vi "PDF Protokoll.vi"(8 "error in (no error)":errorcluster caption="Fehler (Eingang, kein Fehler)") -> (0 "error out":errorcluster caption="Fehler (Ausgang)")   [LabVIEW 2015, in "Linearisierung V2.lvlib" / "Protokoll.lvlib"]
uses:
  Protokoll.lvlib
  EPA Ausgabetabelle.ctl
  AktivArray.ctl
  AktivButton.ctl
  Aktion Lin Daten aufarbeiten.ctl
  EPA1065-307/Aktion FGV Auswertung sammeln.ctl
  <vilib>/Utility/miscctls.llb/LVPrintingMarginsTypeDef.ctl
  Linearisierung V2.lvlib
  EPA1065-307/Linearity verification 1065-307.lvlib
  Allgemein/allgemeine Sub-VIs.lvlib
  <vilib>/Utility/NIReport.llb/NI_ReportGenerationCore.lvlib
panel:
  out "XY-Graph EPA":cluster{dbl[], dbl[]}[](graph) caption="XY-Graph"
  out "Aktiv":T1
  out "EPA Ausgabetabelle":T3
  out "Ergebnis:":string
  out "Konzentration:":string
  out "Komponente:":string
  out "Bearbeiter:":string
  out "Gasteiler:":string
  out "Messgerät:":string
  out "EPA Auswertung":string[][](table) caption="Evaluation"
  # "Linearity Check EPA §1065.307"
  # "Linearity Check EPA § 1065.307"
  # "IAG-Industrie Automatisierungsgeschellschaft m.b.H.    l  Industriestraße 2    l    2722Weikersdorf     )+43262221734 7+43262221734655"
  # "Linearity detection §1065.307"
  # "Description of the limits"
  # "Slope (a1) value between 0,99-1,01"
  # "Intercept (a0)"
  # "laboratory: Value <= 0,5% of the gas concentration"
  # "field: Value <= 1% of the gas concentration"
  # "Coefficient of determination (R²) Value >= 0,998"
  # "standard error of estimate (SEE) Value <= 1% of the gas concentration"
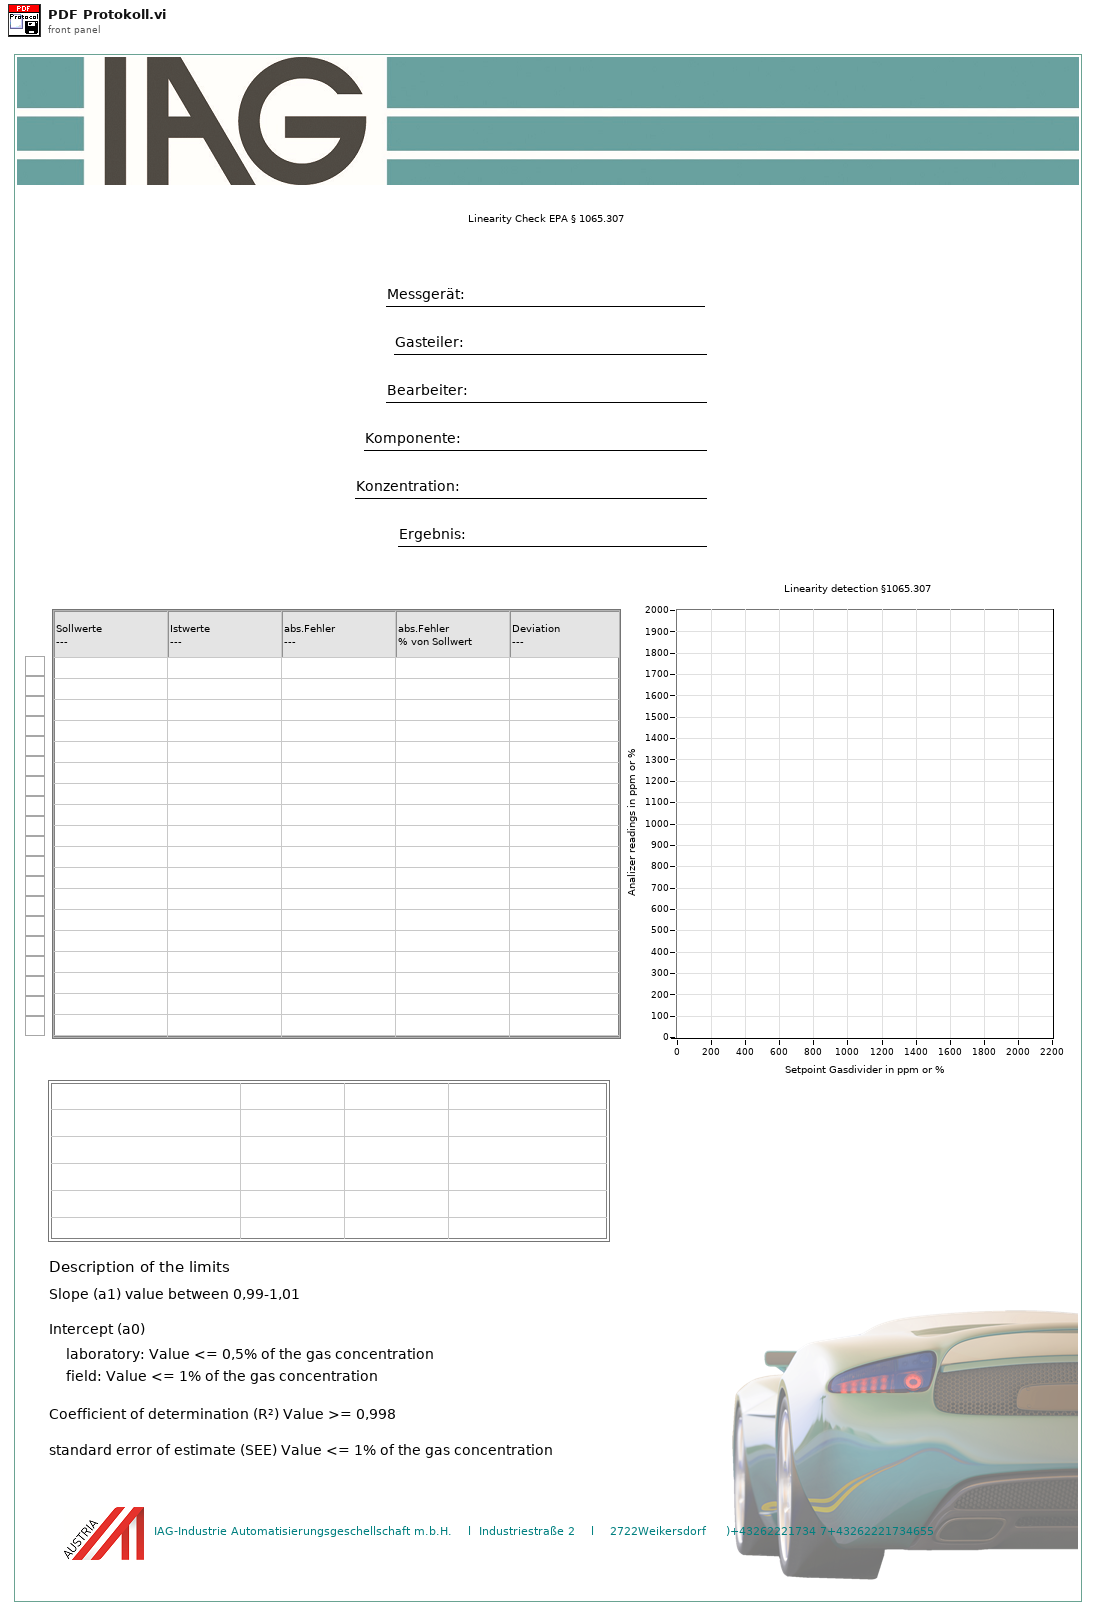
[diagram p1: front panel]
types:
  T1 = typedef "Linearisierung V2.lvlib/AktivArray.ctl" = T2[]
  T2 = typedef "Linearisierung V2.lvlib/AktivButton.ctl" = bool
  T3 = typedef "Linearisierung V2.lvlib/EPA Ausgabetabelle.ctl" = string[][]
  T4 = typedef "Linearisierung V2.lvlib/Aktion Lin Daten aufarbeiten.ctl" = enum16{"lesen", "Protkolldaten", "speichern", "laden", "EPA auswerten", "Tabelle schreiben", "Lin auswerten", "Tab init", "Stufentabelle", "EPA aktiviert", "Nachbehandlung laden", "Tabelle löschen", "Istwerte löschen", "Zeile löschen", "Zeile einfügen", "LIN aktiviert", "LIN/EPA aktiv laden"}
  T5 = typedef "Linearisierung V2.lvlib/Linearity verification 1065-307.lvlib/Aktion FGV Auswertung sammeln.ctl" = enum16{"lesen", "Auswertung", "löschen"}
  T6 = enum32{"Portrait", "Landscape", "Rotated Portrait", "Rotated Landscape"}
  T7 = typedef "LVPrintingMarginsTypeDef.ctl" = cluster{"Top":sgl, "Left":sgl, "Bottom":sgl, "Right":sgl, "Measurement System":enum8{"Inches", "cm"}}
  T8 = typedef "Auswahlfeld.ctl" = u16
  T9 = typedef "Linearisierung V2.lvlib/Eingabetabelle.ctl" = string[][]
  T10 = typedef "Linearisierung V2.lvlib/Lin-Polynom Daten.ctl" = cluster{"Messgerät":string, "Kalibrator (Gasteiler)":string, "Bearbeiter/in":string, "Komponente":string, "Zeitstempel":timestamp, "F_max gefordert (%)":sgl, "F_max in %":sgl, "F_max in ppm":sgl, "Vorschlag Ordnung":i32, "Polynom OK":bool, "Polynomkoeff.":sgl[], "Prüfgas Konzentration":sgl, "Pfad1":string, "Pfad_LIN":string, "Gasnummer:":u8, "Komponentenauswahl":T11, "Verdünnungsgas":T12, "Zeitdauer Stufe":T13, "Anzahl Stufen":T13, "F_max in % EPA":sgl, "F_max in ppm EPA":sgl, "F_max in % LIN":sgl, "F_max in ppm LIN":sgl, "Punkte umkehren":bool, "EPA Optionsfeld":T14, "Autolin Hovacal":T15}
  T11 = typedef "Linearisierung V2.lvlib/KomponentenArray.ctl" = cluster{"Komponente:":T8, "Konzentration":sgl}[]
  T12 = typedef "Linearisierung V2.lvlib/Gasteiler.lvlib/Prüfgas in.ctl" = u16
  T13 = typedef "Zahlen-Eingabefeld.ctl" = sgl
  T14 = typedef "Linearisierung V2.lvlib/EPA Optionsfeld.ctl" = enum32{"Istwert", "Rohwert", "Linearisierter Wert"}
  T15 = typedef "Linearisierung V2.lvlib/Gasteiler.lvlib/HovaCal.lvlib/AutoLin Hovacal.ctl" = enum32{"Keine Auswahl", "Optionsauswahl 1", "Optionsauswahl 2"}
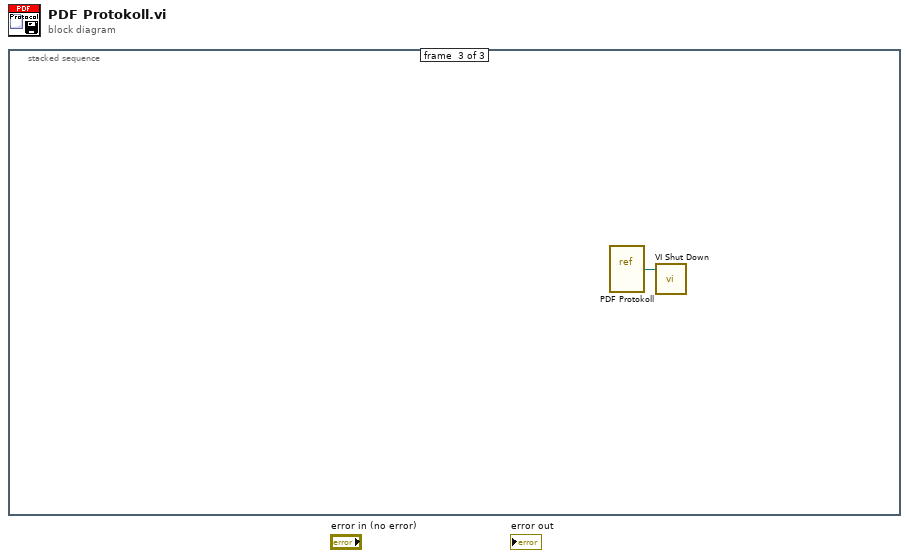
[diagram p0: block diagram]
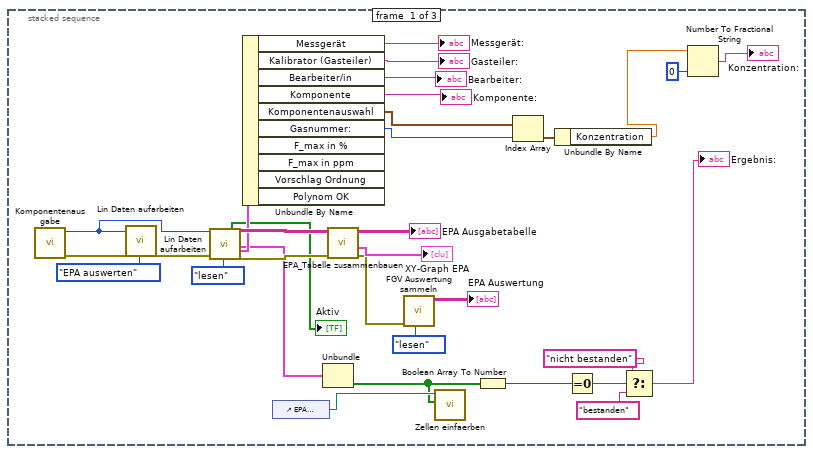
[diagram p2: hidden frame]
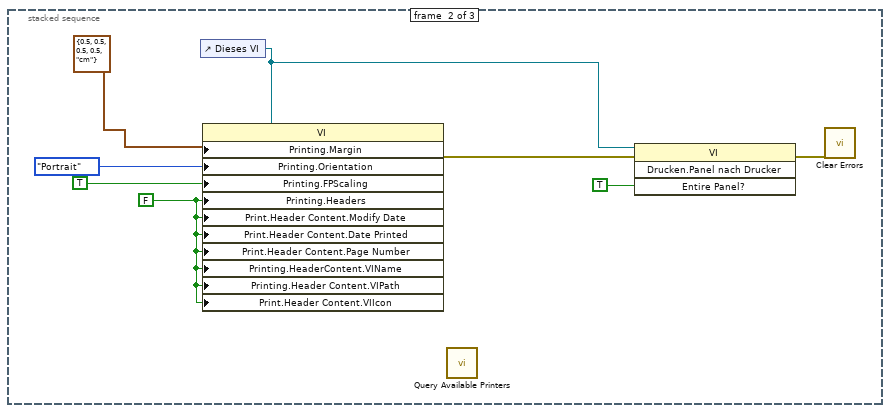
[diagram p3: hidden frame]
diagram:
  n1 = stacked-sequence {
    frame #0 {
      n2 = call "Komponentenausgabe.vi"() -> ("error out"=w7:errorcluster, "Gaskomponente"=w6:T8)  [unwired: 9 in, 1 out]
      n3 = call "Lin Daten aufarbeiten.vi"("Index (Seite)"=w6, "error in (no error)"=w7, "Aktionen"=Aktion_Lin_Daten_aufarbeiten."EPA auswerten") -> ("error out"=w23:errorcluster)  [unwired: 17 in, 7 out]
      n4 = call "Lin Daten aufarbeiten.vi"("Index (Seite)"=w6, "error in (no error)"=w23, "Aktionen"=Aktion_Lin_Daten_aufarbeiten."lesen") -> ("Aktiv EPA"=→"Aktiv":T1, "Eingabetabelle"=w31:T9, "EPA Auswertung"=w15:cluster{sgl[], sgl[], bool[]}, "Lin-Polynom"=w22:T10, "error out"=w30:errorcluster)  [unwired: 17 in, 3 out]
      n5 = Unbundle By Name(w22) -> ("Messgerät"=→"Messgerät:":string, "Kalibrator (Gasteiler)"=→"Gasteiler:":string, "Bearbeiter/in"=→"Bearbeiter:":string, "Komponente"=→"Komponente:":string, "Komponentenauswahl"=w19:T11, "Gasnummer:"=w18:u8)  [unwired: 4 out]
      n6 = control-ref of="EPA Auswertung"() -> (w2:refnum<vi>)
      n7 = Unbundle(w15) -> (w1:bool[])  [unwired: 2 out]
      n8 = call "EPA_Tabelle zusammenbauen.vi"("error in (no error)"=w30, "Eingabetabelle"=w31) -> ("error out"=w26:errorcluster, "XY-Graph"=→"XY-Graph EPA":cluster{dbl[], dbl[]}[], "EPA Ausgabetabelle"=→"EPA Ausgabetabelle":string[][])  [unwired: 7 in]
      n9 = call "FGV Auswertung sammeln.vi"("Aktion"=Aktion_FGV_Auswertung_sammeln."lesen", "error in (no error)"=w26) -> ("LINVer Auswertung"=→"EPA Auswertung":string[][])  [unwired: 8 in, 1 out]
      n10 = call "Zellen einfaerben.vi"("Färben"=w1, "Tabellenref."=w2) -> ()  [unwired: 10 in]
      n11 = Boolean Array To Number(Boolean array=w1) -> (number=w16:u32)
      n12 = Index Array(array=w19, index=w18) -> (element=w17:cluster{"Komponente:":T8, "Konzentration":sgl})
      n13 = Unbundle By Name(w17) -> ("Konzentration"=w9:sgl)
      n14 = Equal To 0?(x=w16) -> (x = 0?=w14:bool)
      n15 = Select(t="nicht bestanden", s=w14, f="bestanden") -> (s? t:f=→"Ergebnis:":string)
      n16 = Number To Fractional String(number=w9, precision (6)=i16 0 ("Genauigkeit (6)")) -> (F-format string=→"Konzentration:":string)  [unwired: 2 in]
    }
    frame #1 {
      w36 = FALSE ("Drucken:Kopfzeilen?")
      n17 = control-ref of="Dieses VI"() -> (w33:refnum<vi>)
      n18 = property class="VI"(reference=w33, "Printing.Margin"=T7 {"Top"=0.5, "Left"=0.5, "Bottom"=0.5, "Right"=0.5, "Measurement System"=enum."cm"} ("Drucken:Ränder"), "Printing.Orientation"=T6."Portrait" ("Drucken:Seitenausrichtung"), "Printing.FPScaling"=TRUE ("Drucken:Frontpanel-Skalierung?"), "Printing.Headers"=w36, "Print.Header Content.Modify Date"=w36, "Print.Header Content.Date Printed"=w36, "Print.Header Content.Page Number"=w36, "Printing.HeaderContent.VIName"=w36, "Printing.Header Content.VIPath"=w36, "Print.Header Content.VIIcon"=w36) -> (error out=w40:errorcluster)  [unwired: 1 in, 1 out]
      n19 = call <vilib>:"Query Available Printers.vi"() -> ()  [unwired: 9 in, 3 out]
      n20 = invoke class="VI" method="Drucken.Panel nach Drucker"(reference=w33, error in=w40, "Entire Panel?"=TRUE ("Abschnittskopfzeilen?")) -> (error out=w34:errorcluster)  [unwired: 1 in, 3 out]
      n21 = call <vilib>:"Clear Errors.vi"("error in (no error)"=w34) -> ()  [unwired: 5 in, 2 out]
    }
    frame #2 {
      n22 = vi-ref "PDF Protokoll.vi"() -> (w41:refnum<vi>)
      n23 = call "VI Shut Down.vi"("VI Referenz"=w41) -> ()  [unwired: 11 in]
    }
  }
